vi "PREOSdll.vi"(8 "error in (no error)":errorcluster, 11 "i":i32) -> (0 "error out":errorcluster)   [LabVIEW 2015]
doc: "subroutine PREOS (i)\n\nTurn on or off the use of the PR cubic equation. Should be called after\ncalling SETUP.\n\nINPUTS:\ni--flag specifying use of PR:\n 0 - Use full equation of state (Peng-Robinson off)\n 1 - Use full equation of state with Peng-Robinson for sat. conditions\n (not currently working)\n 2 - Use Peng-Robinson equation for all calculations\n if i=-1, then i is returned with current usage of PR: 0, 1, or 2."
uses:
  REFPROP.dll
panel:
  # "REFPROP-PREOSdll.vi"
  # "void  PREOSdll(int32_t i);"
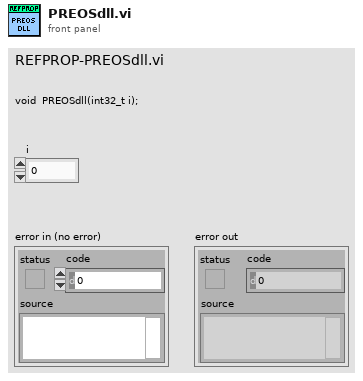
[diagram p1: front panel]
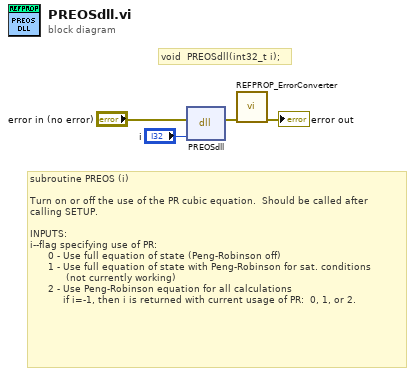
[diagram p0: block diagram]
diagram:
  # "void  PREOSdll(int32_t i);"
  # "subroutine PREOS (i)\n\nTurn on or off the use of the PR cubic equation.  Should be called after\ncalling SETUP.\n\nINPUTS:\ni--flag specifying use of PR:\n      0 - Use full equation of state (Peng-Robinson off)\n      1 - Use full equation of state with Peng-Robinson for sat. conditions\n            (not currently working)\n      2 - Use Peng-Robinson equation for all calculations\n           if i=-1, then i is returned with current usage of PR:  0, 1, or 2."
  n1 = dll-call lib="C:/Users/lauria/Desktop/REFPROP 10 LabVIEW Wrapper BETA/REFPROP/REFPROP.*" fn="PREOSdll"(error in="error in (no error)", "i"="i") -> (error out=w3:errorcluster)  [unwired: 4 in, 1 out]
  n2 = call "REFPROP_ErrorConverter.vi"("error in (no error)"=w3) -> ("error out"=→"error out":errorcluster)  [unwired: 10 in]
